vi "Cnt_OpenConfig.vi"(1 "SampleSettings":T2={"samples per channel"=100, "SampleRate"=1000.0, "TansMaxLength"=500000.0, "ReadTimeOut"=10.0, "时钟源"=""}, 2 "Cnt_ChannelSettings":T1 {"Cnt_ChannelSettings"."decoding type" items=["X1"=10090, "X2"=10091, "X4"=10092, "双脉冲计数"=10313]; "Cnt_ChannelSettings"."z index phase" items=["A High B High"=10040, "A High B Low"=10041, "A Low B High"=10042, "A Low B Low"=10043, ""=0]; "Cnt_ChannelSettings"."单位" items=["Radians"=10273, "Degrees"=10146, "Meters"=10219, "Inches"=10379, "Ticks"=10304, "From Custom Scale"=10065]}, 5 "error In":errorcluster caption="error out") -> (15 "counter_task_out":refnum<k21>[](array[refnum]), 19 "error out":errorcluster)   [LabVIEW 2020, in "NI_DAQ.lvclass"]
uses:
  NI_DAQ.lvclass
  DAQ_Base_class/protected/SampleSettings.ctl
  DAQ_Base_class/protected/Cnt_ChannelSettings.ctl
  <vilib>/DAQmx/create/channels.llb/DAQmx Create Channel (CI-Position-Angular Encoder).vi
  <vilib>/DAQmx/create/channels.llb/DAQmx Create Channel (CI-Position-Linear Encoder).vi
  <vilib>/DAQmx/configure/timing.llb/DAQmx Timing (Sample Clock).vi
  DAQ_Base_class/DAQ_Base.lvclass
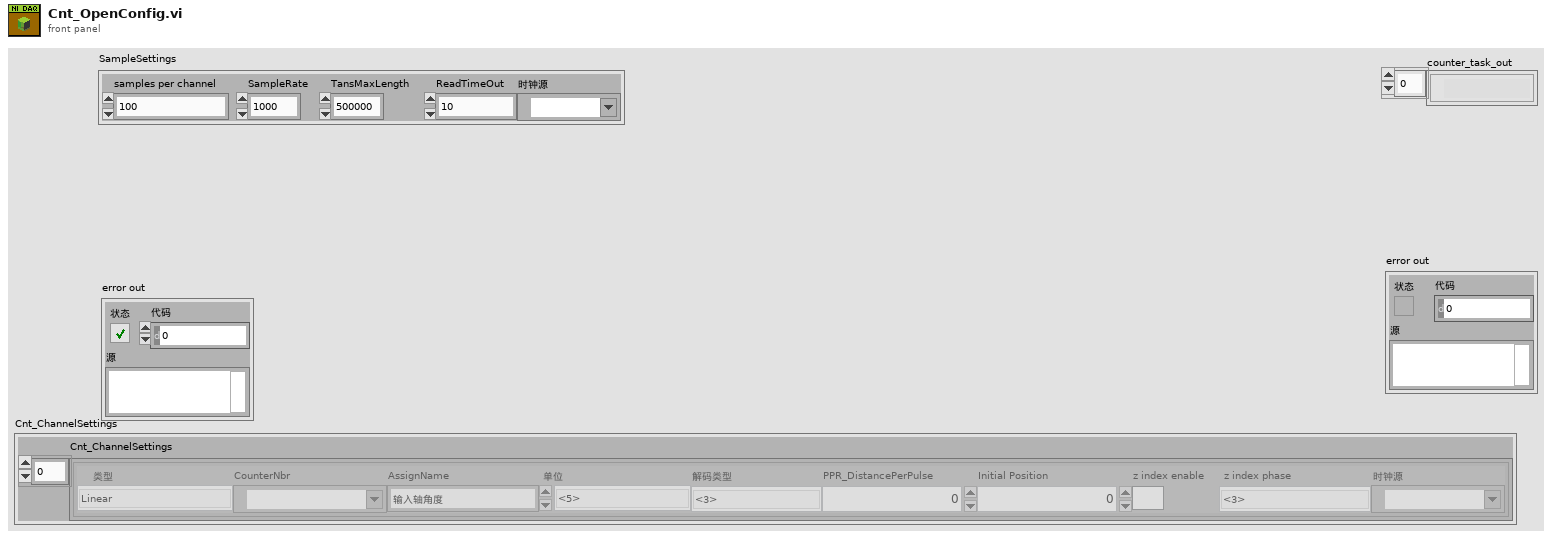
[diagram p1: front panel]
types:
  T1 = typedef "DAQ_Base.lvclass/Cnt_ChannelSettings.ctl" = cluster{"Cnt_ChannelSettings":cluster{"类型":enum16{"Linear", "Rotate"}, "CounterNbr":tag, "AssignName":string, "单位":u16, "decoding type":u16, "PPR_DistancePerPulse":dbl, "Initial Position ":dbl, "z index enable":bool, "z index phase":i32, "source":tag}[]}
  T2 = typedef "DAQ_Base.lvclass/SampleSettings.ctl" = cluster{"samples per channel":i32, "SampleRate":dbl, "TansMaxLength":dbl, "ReadTimeOut":dbl, "时钟源":tag}
  T3 = cluster{"类型":enum16{"Linear", "Rotate"}, "CounterNbr":tag, "AssignName":string, "单位":u16, "decoding type":u16, "PPR_DistancePerPulse":dbl, "Initial Position ":dbl, "z index enable":bool, "z index phase":i32, "source":tag}[]
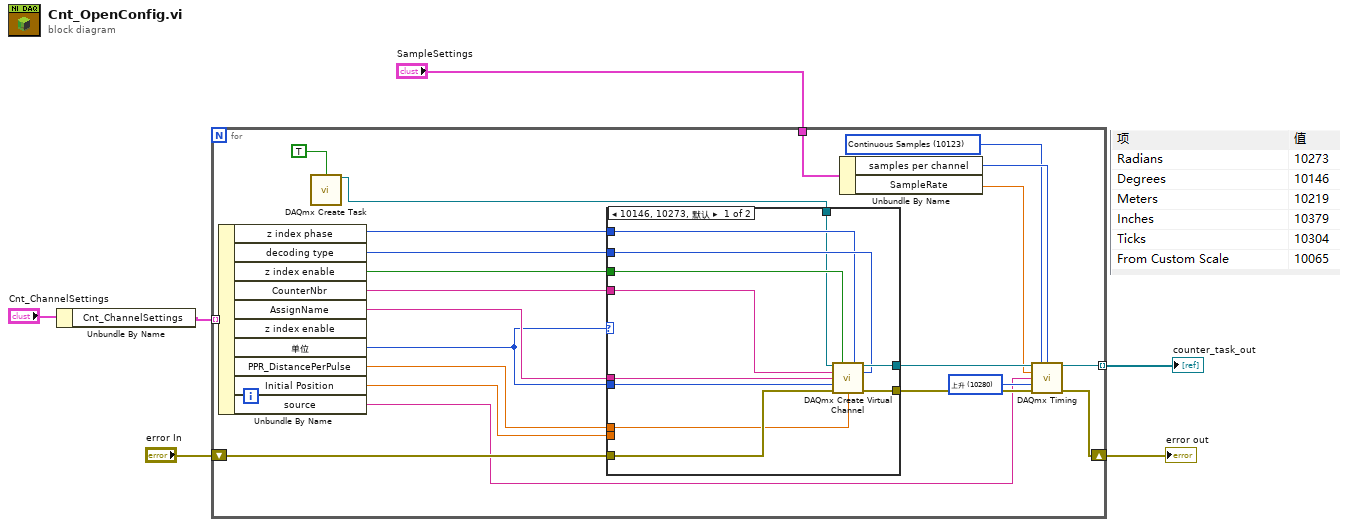
[diagram p0: block diagram]
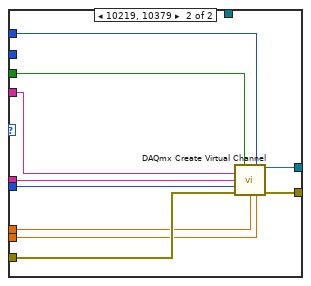
[diagram p2: hidden frame]
diagram:
  n1 = Unbundle By Name("Cnt_ChannelSettings") -> ("Cnt_ChannelSettings"=w1:T3)
  n2 = for {
    shift-right: [w24] -> w5
    shift-left: "error In" -> [w28]
    tunnel: [w26] -> w6 mode=indexing
    tunnel: w1 -> [w19] mode=indexing
    tunnel: "SampleSettings" -> [w11]
    w20 = 10280 items=["上升"=10280, "下降"=10171] ("active edge")
    w21 = 10123 items=["Finite Samples"=10178, "Continuous Samples"=10123, "Hardware Timed Single Point"=12522] ("sample mode")
    n3 = Unbundle By Name(w19) -> ("z index phase"=w16:i32, "decoding type"=w17:u16, "z index enable"=w18:bool, "CounterNbr"=w15:tag, "AssignName"=w14:string, "单位"=w9:u16, "PPR_DistancePerPulse"=w13:dbl, "Initial Position"=w10:dbl, "source"=w12:tag)  [unwired: 1 out]
    n4 = call <vilib>:"DAQmx Create Task.vi"("auto cleanup"=TRUE) -> ("task out"=w7:refnum<k21>)  [unwired: 13 in, 1 out]
    n5 = case shown="10146, 10273, 默认" w9 {
      tunnel: w16 -> [w30 w49]
      tunnel: [w39 w48] -> w27
      tunnel: w28 -> [w38 w47]
      tunnel: [w37 w46] -> w25
      tunnel: w18 -> [w36 w42]
      tunnel: w17 -> [w35 _]
      tunnel: w15 -> [w34 w44]
      tunnel: w14 -> [w33 w43]
      tunnel: w9 -> [w32 w45]
      tunnel: w13 -> [w31 w41]
      tunnel: w10 -> [_ w40]
      tunnel: w7 -> [w29 _]
      frame 10146, 10273, Default {
        n6 = call-poly <vilib>:"DAQmx Create Virtual Channel.vi"("task in"=w29, "z index enable"=w36, "z index phase"=w30, "counter"=w34, "decoding type"=w35, "name to assign"=w33, "units"=w32, "error in"=w38, "pulses per revolution"=w31) -> ("task out"=w39:refnum<k21>, "error out"=w37:errorcluster)  [unwired: 3 in, 2 out]
      }
      frame 10219, 10379 {
        n7 = call-poly <vilib>:"DAQmx Create Virtual Channel.vi"("z index enable"=w42, "z index phase"=w49, "counter"=w44, "name to assign"=w43, "units"=w45, "error in"=w47, "distance per pulse"=w41, "initial position"=w40) -> ("task out"=w48:refnum<k21>, "error out"=w46:errorcluster)  [unwired: 4 in, 2 out]
      }
    }
    n8 = Unbundle By Name(w11) -> ("samples per channel"=w23:i32, "SampleRate"=w22:dbl)
    n9 = call-poly <vilib>:"DAQmx Timing.vi"("task/channels in"=w27, "sample mode"=w21, "samples per channel"=w23, "rate"=w22, "source"=w12, "active edge"=w20, "error in"=w25) -> ("task out"=w26:refnum<k21>, "error out"=w24:errorcluster)  [unwired: 1 in, 6 out]
  }
  "error out" <- w5
  "counter_task_out" <- w6
